vi "AKD Move Rel.vi"(0 "TCP Refnum in":refnum<k5>, 7 "MT ID":u16, 11 "error in":errorcluster) -> (4 "TCP Refnum out":refnum<k5>, 15 "error out":errorcluster)   [LabVIEW 2019]
doc: "This VI will issue a move command to the AKD drive to enact the specific MT.\nNote: the Motion Task ID input must already have a MT initialised - this can be done using AKD Create MT.vi"
uses:
  MODBUS/NI Modbus.llb/MB Ethernet Master Query Write Multiple Registers (poly).vi
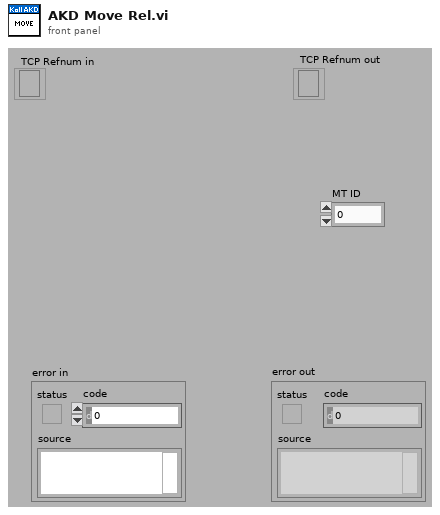
[diagram p1: front panel]
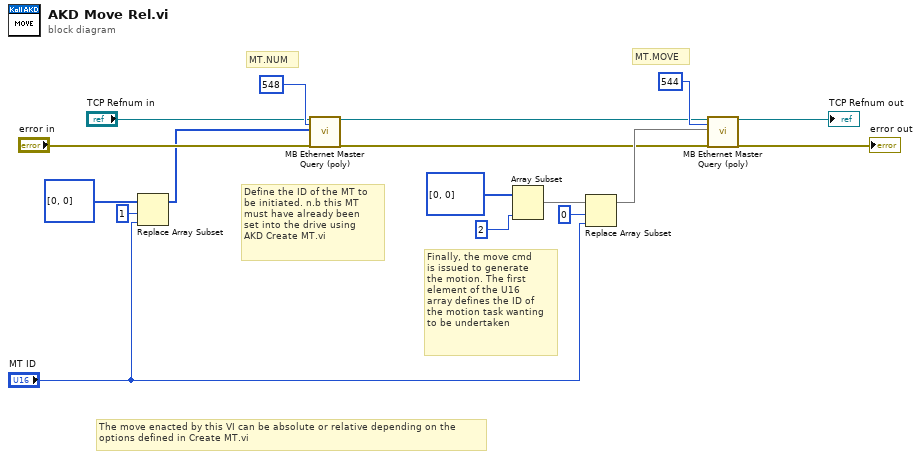
[diagram p0: block diagram]
diagram:
  # "The move enacted by this VI can be absolute or relative depending on the\noptions defined in Create MT.vi"
  # "Define the ID of the MT to \nbe initiated. n.b this MT\nmust have already been \nset into the drive using\nAKD Create MT.vi"
  # "Finally, the move cmd\nis issued to generate\nthe motion. The first\nelement of the U16\narray defines the ID of\nthe motion task wanting\nto be undertaken"
  # "MT.MOVE"
  # "MT.NUM"
  n1 = Replace Array Subset(array=u16[] [0, 0], new element="MT ID", index=1) -> (w9:u16[])
  n2 = call-poly "MB Ethernet Master Query (poly).vi"("TCP Connection Refnum in"="TCP Refnum in", "Starting Address"=u16 548, "Registers"=w9, "error in"="error in") -> ("TCP Connection Refnum (dup)"=w1:refnum<k5>, "error out"=w2:errorcluster)  [unwired: 13 in, 1 out]
  n3 = Array Subset(array=u16[] [0, 0], length=2) -> (w4:u16[])  [unwired: 1 in]
  n4 = Replace Array Subset(array=w4, new element="MT ID", index=0) -> (w3:u16[])
  n5 = call-poly "MB Ethernet Master Query (poly).vi"("TCP Connection Refnum in"=w1, "Starting Address"=u16 544, "Registers"=w3, "error in"=w2) -> ("TCP Connection Refnum (dup)"=→"TCP Refnum out":refnum<k5>, "error out"=→"error out":errorcluster)  [unwired: 13 in, 1 out]
